vi "T7_Write_Float_Register.vi"(0 "Remote IP Address":string="192.168.126.148", 1 "Remote Port":u16=502, 2 "FirstChannel":u16, 3 "error in (no error)":errorcluster, 4 "FLOAT32 to Write":sgl=1.23) -> (9 "WrittenAt":timestamp=timestamp(3513857842.218402 s since 1904-01-01), 10 "error out":errorcluster)   [LabVIEW 2015]
uses:
  Serial Link Layer/NI_Modbus_Cleaned/NI Modbus121Clean.llb/MB Ethernet Master Query Write Multiple Registers (poly).vi
panel:
  out "Starting Address":u16=1002
  # "MB Ethernet Example Master.vi\n\nInstructions\n1.Use Kipling to find your devices IP address & modify the\n\"Remote IP Addres\"\n2. Run this VI\n3. Change value of \"FLOAT32 to Write\" & press \"Write Data\""
  # "TCP Parameters"
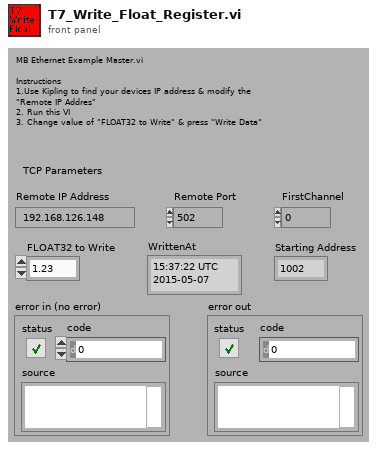
[diagram p1: front panel]
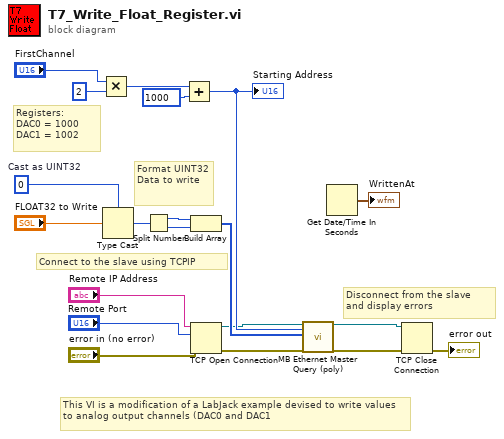
[diagram p0: block diagram]
diagram:
  w10 = u32 0  # Cast as UINT32
  # "This VI is a modification of a LabJack example devised to write values to analog output channels (DAC0 and DAC1"
  # "Format UINT32 Data to write"
  # "Registers:\nDAC0 = 1000\nDAC1 = 1002"
  # "Disconnect from the slave\nand display errors"
  # "Connect to the slave using TCPIP"
  n1 = Multiply(x="FirstChannel", y=u16 2) -> (x*y=w16:u16)
  n2 = Type Cast(type=w10, x="FLOAT32 to Write") -> (*(type *) &x=w9:u32)
  n3 = Split Number(x=w9) -> (hi(x)=w8:u16, lo(x)=w7:u16)
  n4 = Add(x=w16, y=1000) -> (x+y=w6:i32)
  "Starting Address" <- w6
  n5 = Build Array(w8, w7) -> (w12:u16[])
  n6 = TCP Open Connection(address="Remote IP Address", remote port or service name="Remote Port", error in (no error)="error in (no error)") -> (connection ID=w1:refnum<k5>, error out=w2:errorcluster)  [unwired: 2 in]
  n7 = call-poly "MB Ethernet Master Query (poly).vi"("TCP Connection Refnum in"=w1, "Starting Address"=w6, "Registers"=w12, "error in"=w2) -> ("TCP Connection Refnum (dup)"=w4:refnum<k5>, "error out"=w3:errorcluster)  [unwired: 13 in, 1 out]
  n8 = Get Date/Time In Seconds() -> (seconds since 1Jan1904=→"WrittenAt":timestamp)
  n9 = TCP Close Connection(connection ID=w4, error in (no error)=w3) -> (error out=→"error out":errorcluster)  [unwired: 2 out]
